vi "write_sens.vi"(8 "error in (no error)":errorcluster, 11 "Sens":dbl=10000.0 format="%#_13g") -> (0 "error out":errorcluster)   [LabVIEW 2019, in "NEXUS.lvclass"]
uses:
  NEXUS.lvclass
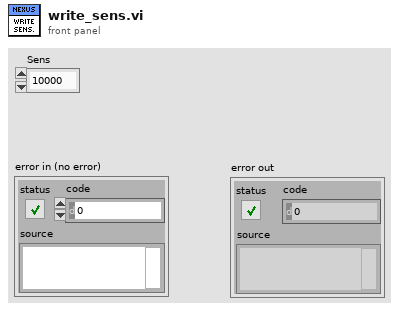
[diagram p1: front panel]
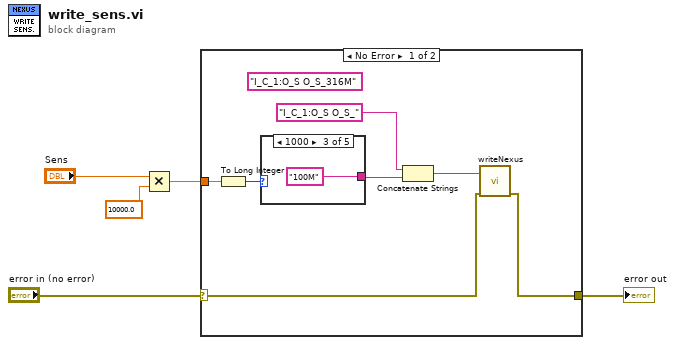
[diagram p0: block diagram]
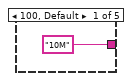
[diagram p2: hidden frame]
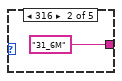
[diagram p3: hidden frame]
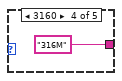
[diagram p4: hidden frame]
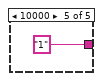
[diagram p5: hidden frame]
diagram:
  n1 = Multiply(x="Sens", y=10000.0) -> (x*y=w4:dbl)
  n2 = case shown="No Error" "error in (no error)" {
    selector: "error in (no error)" -> [w7 w18]
    tunnel: w4 -> [w9 _]
    tunnel: [w6 w18] -> w1
    frame No Error {
      (unwired) "I_C_1:O_S O_S_316M" ("Command")
      n3 = To Long Integer(number=w9) -> (32bit integer=w12:i32)
      n4 = case shown="1000" w12 {
        tunnel: ["10M" ("Command") "31_6M" ("Command") "100M" ("Command") "316M" ("Command") "1" ("Command")] -> w10
        frame 100, Default {
        }
        frame 316 {
        }
        frame 1000 {
        }
        frame 3160 {
        }
        frame 10000 {
        }
      }
      n5 = Concatenate Strings("I_C_1:O_S O_S_" ("Command"), w10) -> (w8:string)
      n6 = call "writeNexus.vi"("error in (no error)"=w7, "Command"=w8) -> ("error out"=w6:errorcluster)  [unwired: 8 in, 1 out]
    }
    frame Error {
    }
  }
  "error out" <- w1
